vi "TempLogger_FilePrompt.vi"() -> (2 "selected path":path, 3 "not cancelled":bool)   [LabVIEW 2022 SP3]
panel:
  out "error out":errorcluster
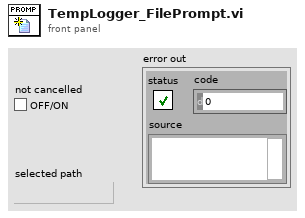
[diagram p1: front panel]
types:
  T1 = enum16{"open", "replace", "create", "open or create", "replace or create", "replace or create with confirmation"}
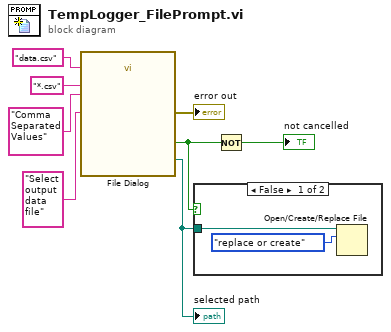
[diagram p0: block diagram]
diagram:
  n1 = call "File Dialog"("prompt"="Select output data file", "default name"="data.csv", "pattern (all files)"="*.csv", "pattern label"="Comma Separated Values") -> ("selected path"=w3:path, "cancelled"=w4:bool, "error out"=→"error out":errorcluster)  [unwired: 8 in, 1 out]
  "selected path" <- w3
  n2 = case shown="False" w4 {
    tunnel: w3 -> [w10 _]
    frame False {
      n3 = Open/Create/Replace File(file path (use dialog)=w10, operation (0:open)=T1."replace or create") -> ()  [unwired: 4 in, 3 out]
    }
    frame True {
    }
  }
  n4 = Not(x=w4) -> (.not. x?=→"not cancelled":bool)
